vi "WriteVerify Mfg Serial Number.vi"(8 "error in":errorcluster, 11 "Serial Number":string) -> (0 "error out":errorcluster)   [LabVIEW 2015]
panel:
  out "Written Serial Number":string
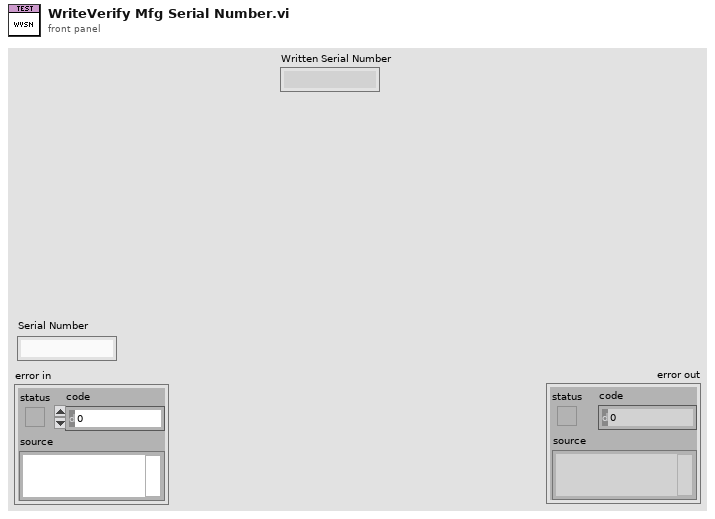
[diagram p1: front panel]
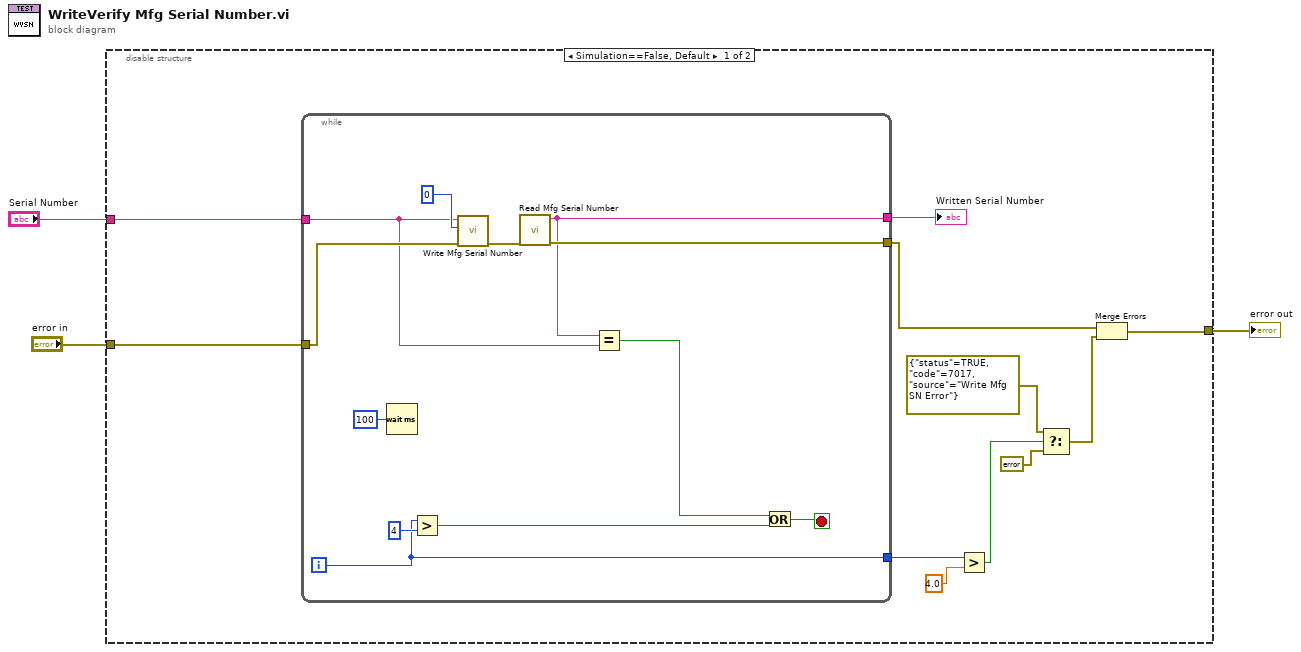
[diagram p0: block diagram]
diagram:
  n1 = disable-structure shown="Simulation==False, Default" {
    disable-tunnel: "error in" -> [w14 w27]
    disable-tunnel: [w5 w27] -> w2
    disable-tunnel: "Serial Number" -> [w13 _]
    frame condition #0 (active) {
      n2 = while {
        tunnel: w14 -> [w18]
        tunnel: w13 -> [w17]
        tunnel: [w19] -> w6
        tunnel: [w22] -> w11
        tunnel: [w15] -> w4
        i -> [w22]
        stop <- w24 stop-if-true
        n3 = Wait (ms)(milliseconds to wait=u32 100) -> ()  [unwired: 1 out]
        n4 = Greater?(x=w22, y=4) -> (0:w25:bool)
        n5 = call "Write Mfg Serial Number.vi"("error in"=w18, "Start Address"=u8 0, "Serial Number"=w17) -> ("error out"=w20:errorcluster)  [unwired: 8 in]
        n6 = call "Read Mfg Serial Number.vi"("error in"=w20) -> ("error out"=w19:errorcluster, "Serial Number"=w15:string)  [unwired: 9 in]
        n7 = Equal?(x=w15, y=w17) -> (x = y?=w16:bool)
        n8 = Or(x=w16, y=w25) -> (x .or. y?=w24:bool)
      }
      "Written Serial Number" <- w4
      n9 = Greater?(x=w11, y=4.0) -> (0:w10:bool)
      n10 = Select(t=errorcluster {"status"=TRUE, "code"=7017, "source"="Write Mfg SN Error"} ("f"), s=w10, f=errorcluster {"status"=FALSE, "code"=0, "source"=""}) -> (s? t:f=w7:errorcluster)
      n11 = Merge Errors(w6, w7) -> (w5:errorcluster)
    }
    frame condition #1 {
    }
  }
  "error out" <- w2
